vi "CameraTempControllerRunner.vi"(8 "error in (no error)":errorcluster, 9 "tempControllerBackEndEvents in":T1, 10 "tempControllerFrontEndEvents in":T2, 11 "CameraTempController":refnum<class "CameraTempController.lvclass">) -> (0 "error out":errorcluster, 1 "tempControllerBackEndEvents out":T1, 2 "tempControllerFrontEndEvents out":T2, 3 "CameraTempController out":refnum<class "CameraTempController.lvclass">)   [LabVIEW 2011, in "Hardware.lvlib" / "Channels.lvlib" / "CameraTempControllerRunner.lvclass"]
uses:
  CameraTempControllerRunner.lvclass
  CameraTempController.lvclass
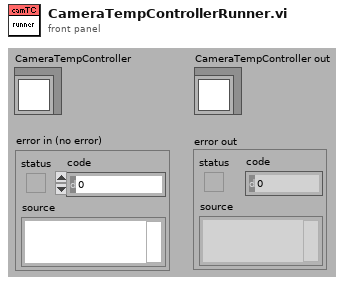
[diagram p1: front panel]
types:
  T1 = cluster{"closeEvent":refnum<user-event>, "temperatureUpdateEvent":refnum<user-event>, "displayErrorEvent":refnum<user-event>, "setPointUpdateEvent":refnum<user-event>}
  T2 = cluster{"newSetPointEvent":refnum<user-event>, "stopCoolingEvent":refnum<user-event>}
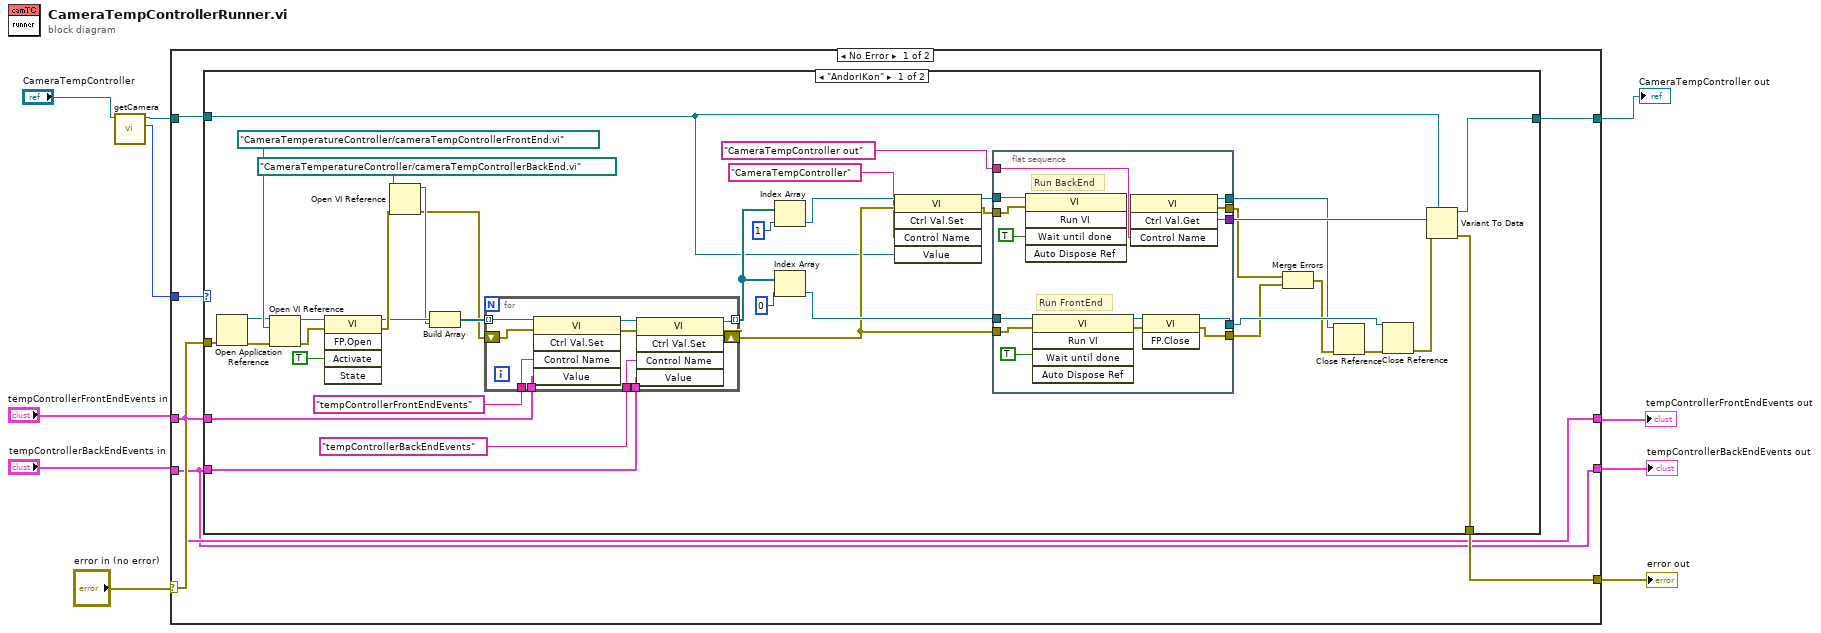
[diagram p0: block diagram]
diagram:
  n1 = call-dynamic "getCamera.vi"("CameraTempController.lvclass in"="CameraTempController") -> ("Camera"=w1:enum16{"AndorIKon", "ICCamera"}, "CameraTempController.lvclass out"=w2:refnum<class "CameraTempController.lvclass">)  [unwired: 8 in, 1 out]
  n2 = case shown="No Error" "error in (no error)" {
    selector: "error in (no error)" -> [w14 w87]
    tunnel: [w16 w87] -> w9
    tunnel: w2 -> [w17 w86]
    tunnel: [w15 w86] -> w8
    tunnel: "tempControllerFrontEndEvents in" -> [w13 w85]
    tunnel: "tempControllerBackEndEvents in" -> [w12 w84]
    tunnel: [w13 w85] -> w5
    tunnel: [w12 w84] -> w4
    tunnel: w1 -> [w11 _]
    frame No Error {
      n3 = case shown="\"AndorIKon\"" w11 {
        tunnel: w17 -> [w31 w83]
        tunnel: [w30 w82] -> w16
        tunnel: [w28 w83] -> w15
        tunnel: w14 -> [w20 w82]
        tunnel: w13 -> [w19 _]
        tunnel: w12 -> [w18 _]
        frame "AndorIKon" {
          n4 = Open Application Reference(8:w20) -> (0:w50:errorcluster, 3:w52:refnum<vi>)  [unwired: 3 in]
          n5 = Open VI Reference(application reference (local)=w52, vi path=path "CameraTemperatureController/cameraTempControllerFrontEnd.vi", error in (no error)=w50) -> (vi reference=w54:refnum<vi>, error out=w51:errorcluster)  [unwired: 3 in]
          n6 = invoke class="VI" method="FP.Open"(reference=w54, error in=w51, "Activate"=TRUE) -> (reference out=w47:refnum<vi>, error out=w49:errorcluster)  [unwired: 2 in, 3 out]
          n7 = Open VI Reference(vi path=path "CameraTemperatureController/cameraTempControllerBackEnd.vi", error in (no error)=w49) -> (vi reference=w40:refnum<vi>, error out=w39:errorcluster)  [unwired: 4 in]
          n8 = Build Array(w47, w40) -> (w46:refnum<vi>[])
          n9 = for {
            tunnel: "tempControllerFrontEndEvents" -> [w81]
            tunnel: [w77] -> w43 mode=indexing
            tunnel: w46 -> [w80] mode=indexing
            shift-right: [w78] -> w35
            shift-left: w39 -> [w79]
            tunnel: w19 -> [w74]
            tunnel: "tempControllerBackEndEvents" -> [w73]
            tunnel: w18 -> [w72]
            n10 = invoke class="VI" method="Ctrl Val.Set"(reference=w80, error in=w79, "Control Name"=w81, "Value"=w74) -> (reference out=w76:refnum<vi>, error out=w75:errorcluster)  [unwired: 1 in, 3 out]
            n11 = invoke class="VI" method="Ctrl Val.Set"(reference=w76, error in=w75, "Control Name"=w73, "Value"=w72) -> (reference out=w77:refnum<vi>, error out=w78:errorcluster)  [unwired: 1 in, 3 out]
          }
          n12 = Index Array(array=w43, index=1) -> (element=w41:refnum<vi>)
          n13 = Index Array(array=w43, index=0) -> (element=w44:refnum<vi>)
          n14 = invoke class="VI" method="Ctrl Val.Set"(reference=w41, error in=w35, "Control Name"="CameraTempController", "Value"=w31) -> (reference out=w38:refnum<vi>, error out=w37:errorcluster)  [unwired: 1 in, 3 out]
          n15 = flat-sequence {
            tunnel: w44 -> [w70]
            tunnel: w38 -> [w65]
            tunnel: w37 -> [w64]
            tunnel: w35 -> [w68]
            tunnel: [w56] -> w34
            tunnel: [w57] -> w25
            tunnel: "CameraTempController out" -> [w66]
            tunnel: [w67] -> w32
            tunnel: [w60] -> w26
            tunnel: [w61] -> w29
            frame #0 {
              # "Run BackEnd"
              # "Run FrontEnd"
              n16 = invoke class="VI" method="Run VI"(reference=w65, error in=w64, "Wait until done"=TRUE) -> (reference out=w62:refnum<vi>, error out=w63:errorcluster)  [unwired: 2 in, 3 out]
              n17 = invoke class="VI" method="Run VI"(reference=w70, error in=w68, "Wait until done"=TRUE) -> (reference out=w58:refnum<vi>, error out=w59:errorcluster)  [unwired: 2 in, 3 out]
              n18 = invoke class="VI" method="Ctrl Val.Get"(reference=w62, error in=w63, "Control Name"=w66) -> (reference out=w61:refnum<vi>, error out=w60:errorcluster, "Get Control Value Variant"=w67:variant)  [unwired: 1 in, 1 out]
              n19 = invoke class="VI" method="FP.Close"(reference=w58, error in=w59) -> (reference out=w56:refnum<vi>, error out=w57:errorcluster)  [unwired: 1 in, 1 out]
            }
          }
          n20 = Merge Errors(w26, w25) -> (w24:errorcluster)
          n21 = Close Reference(reference=w29, error in (no error)=w24) -> (error out=w36:errorcluster)
          n22 = Close Reference(reference=w34, error in (no error)=w36) -> (error out=w21:errorcluster)
          n23 = Variant To Data(error in=w21, type=w31, Variant=w32) -> (data=w28:refnum<class "CameraTempController.lvclass">, error out=w30:errorcluster)
        }
        frame "ICCamera", Default {
        }
      }
    }
    frame Error {
    }
  }
  "error out" <- w9
  "CameraTempController out" <- w8
  "tempControllerFrontEndEvents out" <- w5
  "tempControllerBackEndEvents out" <- w4
